vi "SimpleExample.vi"(8 "error in (no error)":errorcluster) -> (0 "error out":errorcluster)   [LabVIEW 2014]
uses:
  TableLogger_Actor/TableLoggerConfig.ctl
  TableLogger_Actor/TableLoggerTypes.ctl
  TableLogger_Actor/TableLoggerBackupConfig.ctl
  TableLogger_Actor/Messages/InsertData_Msg/InsertData Msg.lvclass/InsertData Msg.ctl
  <vilib>/ActorFramework/Message Enqueuer/Message Enqueuer.lvclass/Message Enqueuer.ctl
  <vilib>/ActorFramework/Message Enqueuer/Enqueue.vi
  <vilib>/ActorFramework/Message Priority Queue/Priority Enqueue.vi
  TableLogger_Actor/Messages/InsertData_Msg/InsertData Msg.lvclass
  <vilib>/ActorFramework/Stop Msg/Stop Msg.lvclass
  TableLogger_Actor/TableLogger_Actor/TableLogger_Actor.lvclass
  TableLogger_Actor/TableLogger_Actor.lvlib
panel:
  # "Look at the block diagram for details about this VI"
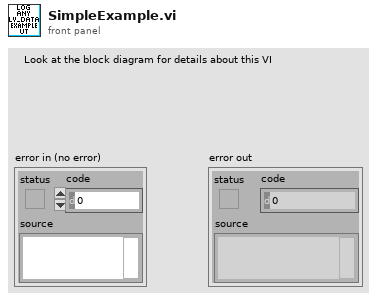
[diagram p1: front panel]
types:
  T1 = typedef "TableLogger_Actor.lvlib/TableLoggerConfig.ctl" = cluster{"TableLogger":T2, "DB File Path":path, "DB Backup Config":T3}
  T2 = typedef "TableLogger_Actor.lvlib/TableLoggerTypes.ctl" = enum16{"CSV Logger", "SQLite Logger"}
  T3 = typedef "TableLogger_Actor.lvlib/TableLoggerBackupConfig.ctl" = cluster{"Directory":path, "UTC Time Format":bool, "On Launch":bool, "Interval (Hours)":dbl, "Size Multiples (Bytes)":i32}
  T4 = cluster{"Test Start Timestamp":timestamp, "Test End Timestamp":timestamp, "Test Jig Location":string, "Location Time Offset":string, "Test Jig ID":string, "Test Jig Fluid":enum16{"Liquid", "Gas"}, "Test Jig Flow":enum16{"Low", "High"}, "Control Board SN":string, "Site Number":i32, "Operator ID":string, "Operation Number":string, "DUT Serial Number":string, "DUT Product Number":string, "DUT Flow Range":i32, "DUT FW Revision":string, "DUT TP1 Offset":dbl, "DUT TP2 Offset":dbl, "DUT Cut Off1":dbl, "DUT Cut Off2":dbl, "PreCal Flow Meas":cluster{"FC Flow Set":dbl, "FM Flow Measure":dbl, "UUT Data":dbl}[], "PostCal Flow Meas":cluster{"FC Flow Set":dbl, "FM Flow Measure":dbl, "UUT Data":dbl}[], "DUT_Coeff":dbl[], "DUT_Flow_Error":dbl[], "Calibration Result":enum16{"Pass", "Fail"}}
  T5 = cluster{"Numeric Data":i32, "Float Data":dbl, "String Data":string, "Enum Data":enum16{"Enum Item 1", "Enum Item 2"}, "Array Data":i32[]}
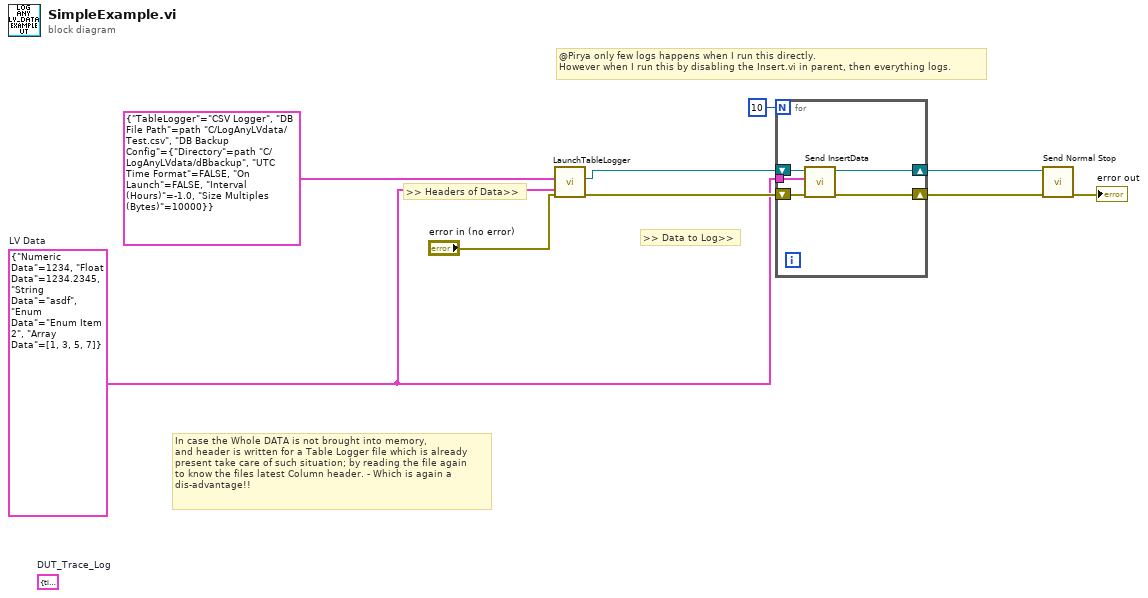
[diagram p0: block diagram]
diagram:
  (unwired) T4 {"Test Start Timestamp"=timestamp(0 s since 1904-01-01), "Test End Timestamp"=timestamp(0 s since 1904-01-01), "Test Jig Location"="asdf", "Location Time Offset"="wer", "Test Jig ID"="xcv", "Test Jig Fluid"=enum."Gas", "Test Jig Flow"=enum."High", "Control Board SN"="fgh", "Site Number"=23, "Operator ID"="op", "Operation Number"="op", "DUT Serial Number"="dt", "DUT Product Number"="dt", "DUT Flow Range"=23, "DUT FW Revision"="asdf", "DUT TP1 Offset"=24.0, "DUT TP2 Offset"=546.0, "DUT Cut Off1"=34.0, "DUT Cut Off2"=453.0, "PreCal Flow Meas"=[{"FC Flow Set"=1.0, "FM Flow Measure"=0.0, "UUT Data"=0.0}, {"FC Flow Set"=2.0, "FM Flow Measure"=0.0, "UUT Data"=0.0}, {"FC Flow Set"=3.0, "FM Flow Measure"=0.0, "UUT Data"=0.0}], "PostCal Flow Meas"=[{"FC Flow Set"=1.0, "FM Flow Measure"=0.0, "UUT Data"=0.0}, {"FC Flow Set"=2.0, "FM Flow Measure"=0.0, "UUT Data"=0.0}], "DUT_Coeff"=[1.0, 2.0], "DUT_Flow_Error"=[1.0, 2.0], "Calibration Result"=enum."Fail"}  # DUT_Trace_Log
  w2 = T5 {"Numeric Data"=1234, "Float Data"=1234.2345, "String Data"="asdf", "Enum Data"=enum."Enum Item 2", "Array Data"=[1, 3, 5, 7]}  # LV Data
  # "In case the Whole DATA is not brought into memory,\nand header is written for a Table Logger file which is already\npresent take care of such situation; by reading the file again\nto know the files latest Column header. - Which is again a \ndis-advantage!!"
  # "@Pirya only few logs happens when I run this directly.\nHowever when I run this by disabling the Insert.vi in parent, then everything logs."
  # ">> Headers of Data>>"
  # ">> Data to Log>>"
  n1 = call "LaunchTableLogger.vi"("error in (no error)"="error in (no error)", "Data Cluster (for Headers)"=w2, "TableLogger Config"=T1 {"TableLogger"=enum."CSV Logger", "DB File Path"=path "C:/LogAnyLVdata/Test.csv", "DB Backup Config"={"Directory"=path "C:/LogAnyLVdata/dBbackup", "UTC Time Format"=FALSE, "On Launch"=FALSE, "Interval (Hours)"=-1.0, "Size Multiples (Bytes)"=10000}}) -> ("error out"=w7:errorcluster, "TableLogger Actor's Enqueuer"=w9:refnum<class "Message Enqueuer.lvclass">)  [unwired: 5 in, 2 out]
  n2 = for {
    N: 10 -> [_]
    tunnel: w2 -> [w12]
    shift-right: [w10] -> w4
    shift-left: w9 -> [w14]
    shift-right: [w11] -> w3
    shift-left: w7 -> [w13]
    n3 = call "Send InsertData.vi"("error in (no error)"=w13, "Data"=w12, "Message Enqueuer"=w14) -> ("error out"=w11:errorcluster, "Message Enqueuer out"=w10:refnum<class "Message Enqueuer.lvclass">)  [unwired: 7 in]
  }
  n4 = call <vilib>:"Send Normal Stop.vi"("error in (no error)"=w3, "Message Enqueuer"=w4) -> ("error out"=→"error out":errorcluster)  [unwired: 9 in]
